vi "Toggle Relay.vi"(8 "error in":errorcluster, 9 "Relay State":bool, 10 "Relay Name":string, 11 "2575 in":refnum<class "2575.lvclass">) -> (0 "error out":errorcluster, 3 "2575 out":refnum<class "2575.lvclass">)   [LabVIEW 2019, in "2575.lvlib" / "2575.lvclass"]
doc: "Set one relay state to either on or off."
uses:
  Library/2575.lvclass
  builds/Instruments/SwitchMatrix.lvlibp/Library/SwitchMatrix.lvclass
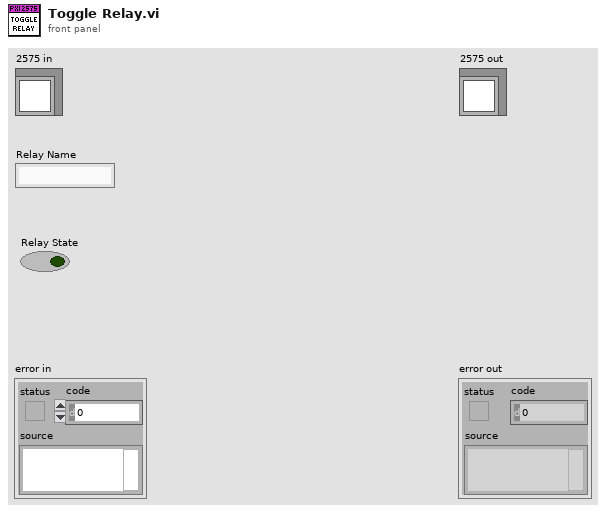
[diagram p1: front panel]
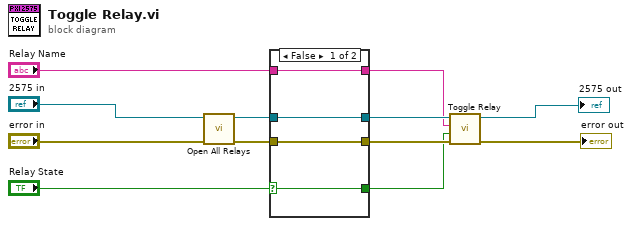
[diagram p0: block diagram]
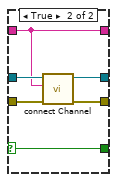
[diagram p2: hidden frame]
diagram:
  n1 = call-dynamic "Open All Relays.vi"("error in"="error in", "2575 in"="2575 in") -> ("error out"=w7:errorcluster, "2575 out"=w8:refnum<class "2575.lvclass">)  [unwired: 8 in]
  n2 = case shown="False" "Relay State" {
    selector: "Relay State" -> [w13 w18]
    tunnel: w8 -> [w16 w22]
    tunnel: [w16 w21] -> w6
    tunnel: [w15 w20] -> w5
    tunnel: w7 -> [w15 w19]
    tunnel: "Relay Name" -> [w14 w17]
    tunnel: [w13 w18] -> w2
    tunnel: [w14 w17] -> w1
    frame False {
    }
    frame True {
      n3 = call "connect Channel.vi"("error in (no error)"=w19, "Channel Name"=w17, "2575 in"=w22) -> ("error out"=w20:errorcluster, "2575 out"=w21:refnum<class "2575.lvclass">)  [unwired: 7 in]
    }
  }
  n4 = call-parent "Toggle Relay.vi"("error in"=w5, "Relay State"=w2, "Relay Name"=w1, "SwitchMatrix in"=w6) -> ("error out"=→"error out":errorcluster, "SwitchMatrix out"=→"2575 out":refnum<class "2575.lvclass">)  [unwired: 6 in]
